vi "acceptMode.vi"(8 "error in (no error)":errorcluster, 10 "Mode Controls":T1, 11 "SR430Class in":refnum<class "SR430Class.lvclass">) -> (0 "error out":errorcluster, 3 "SR430Class out":refnum<class "SR430Class.lvclass">)   [LabVIEW 2015, in "SR430Class.lvclass"]
uses:
  class/SR430Class.lvclass
  class/SR430Class.lvclass/SR430Class.ctl
  support/SR430 Driver/SR430Driver.lvlib
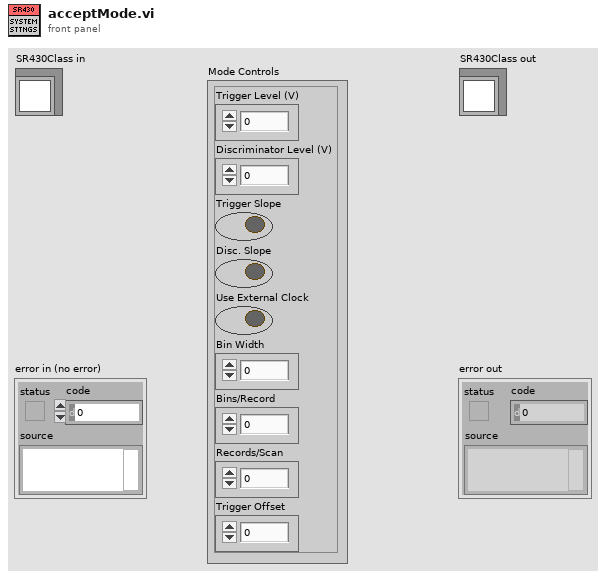
[diagram p1: front panel]
types:
  T1 = cluster{"Trigger Level (V)":dbl, "Discriminator Level (V)":dbl, "Trigger Slope":bool, "Disc. Slope":bool, "Use External Clock":bool, "Bin Width":i32, "Bins/Record":i32, "Records/Scan":i32, "Trigger Offset":i32}
  T2 = typedef "SR430Driver.lvlib/SR430_VISA Control.ctl" = cluster{"VISA resource name":refnum<visa-resource-name>}
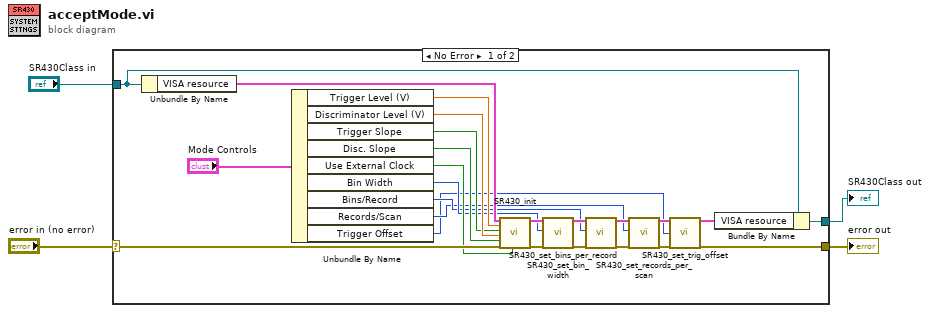
[diagram p0: block diagram]
diagram:
  n1 = case shown="No Error" "error in (no error)" {
    selector: "error in (no error)" -> [w19 w30]
    tunnel: [w6 w30] -> w3
    tunnel: [w20 w29] -> w1
    tunnel: "SR430Class in" -> [w21 w29]
    frame No Error {
      n2 = Unbundle By Name(w21) -> ("VISA resource"=w25:T2)
      n3 = Unbundle By Name("Mode Controls") -> ("Trigger Level (V)"=w17:dbl, "Discriminator Level (V)"=w16:dbl, "Trigger Slope"=w15:bool, "Disc. Slope"=w14:bool, "Use External Clock"=w13:bool, "Bin Width"=w12:i32, "Bins/Record"=w11:i32, "Records/Scan"=w10:i32, "Trigger Offset"=w5:i32)
      n4 = call "SR430_init.vi"("GPIB address"=w25, "triggeLevel [V]"=w17, "triggerSlope"=w15, "discriminatorLevel [V]"=w16, "discriminatorSlope"=w14, "error in (no error)"=w19, "useExternalClock"=w13) -> ("GPIB address out"=w24:T2, "error out"=w28:errorcluster)  [unwired: 11 in]
      n5 = call "SR430_set_bin_width.vi"("address"=w24, "binWidth"=w12, "error in (no error)"=w28) -> ("address out"=w23:T2, "error out"=w27:errorcluster)  [unwired: 15 in]
      n6 = call "SR430_set_bins_per_record.vi"("address"=w23, "binsPerRecord"=w11, "error in (no error)"=w27) -> ("address out"=w22:T2, "error out"=w26:errorcluster)  [unwired: 15 in]
      n7 = call "SR430_set_records_per_scan.vi"("address string"=w22, "recordsPerScan"=w10, "error in (no error)"=w26) -> ("address out"=w9:T2, "error out"=w7:errorcluster)  [unwired: 15 in]
      n8 = call "SR430_set_trig_offset.vi"("address"=w9, "triggerOffset"=w5, "error in (no error)"=w7) -> ("address out"=w8:T2, "error out"=w6:errorcluster)  [unwired: 15 in]
      n9 = Bundle By Name(cluster=w21, "VISA resource"=w8) -> (w20:refnum<class "SR430Class.lvclass">)
    }
    frame Error {
    }
  }
  "error out" <- w3
  "SR430Class out" <- w1
